vi "Tourner_Gyros.vi"(8 "Right":dbl, 9 "Left":dbl, 11 "Angle Voulu":dbl) -> (2 "Angle Reel":dbl)   [LabVIEW 2015]
uses:
  <vilib>/Rock Robotics/WPI/Utilities/WPI_GetSetVariantRefNum.vi
  <vilib>/Rock Robotics/Network Tables/NT Write Number.vi
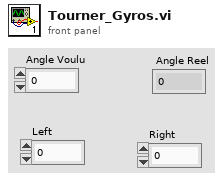
[diagram p1: front panel]
types:
  T1 = typedef "WPI_GyroDevRef.ctl" = cluster{"DevStatus":errorcluster, "Analog Channel":T2, "Offset":dbl, "Gain (VoltsPerDegree/Second)":dbl, "Gyro Type":enum16{"Analog", "XRS450"}, "Handle":i32, "SPI Bus":T3, "Device Found":bool, "Sample Rate":dbl, "Calibrate On Open":bool}
  T2 = typedef "FPGA_AIChannel.ctl" = enum8{"AI 0", "AI 1", "AI 2", "AI 3", "AI MXP 0", "AI MXP 1", "AI MXP 2", "AI MXP 3", "Invalid"}
  T3 = typedef "spi_bus.ctl" = enum16{"SPI On-Board, CS0", "SPI On-Board, CS1", "SPI On-Board, CS2", "SPI On-Board, CS3", "SPI MXP", "Invalid"}
  T4 = typedef "WPI_RobotDriveDevRef.ctl" = cluster{"DevStatus":errorcluster, "Motors[]":T5[], "Square Inputs":bool, "Max Output":dbl}
  T5 = typedef "WPI_MotorControlDeviceRef.ctl" = cluster{"DeviceStatus":errorcluster, "Type":T6, "PWM":cluster{"PWM Channel":T7, "DeadBand":T8}, "CAN":cluster{"Device Number":u8, "Control Mode":T9, "Semaphore":T10, "Max Vout":dbl, "TalonSRX Control Mode":T11}, "Invert":bool}
  T6 = typedef "WPI_MotorControlType.ctl" = enum16{"PWM", "CAN", "CANTalonSRX"}
  T7 = typedef "FPGA_DIOPWMChannel.ctl" = enum8{"PWM 0", "PWM 1", "PWM 2", "PWM 3", "PWM 4", "PWM 5", "PWM 6", "PWM 7", "PWM 8", "PWM 9", "PWM MXP 0", "PWM MXP 1", "PWM MXP 2", "PWM MXP 3", "PWM MXP 4", "PWM MXP 5", "PWM MXP 6", "PWM MXP 7", "PWM MXP 8", "PWM MXP 9", "Invalid"}
  T8 = typedef "WPI_PWMDeadband.ctl" = cluster{"Name":string, "maxPositivePwm":i32, "minPositivePwm":i32, "centerPwm":i32, "maxNegativePwm":i32, "minNegativePwm":i32, "angularRange":u16}
  T9 = typedef "WPI_CANJaguar_ControlMode.ctl" = enum8{"Percent VBus", "Current", "Speed", "Position", "Voltage"}
  T10 = typedef "Semaphore RefNum" = refnum<k1>
  T11 = typedef "WPI_CANTalonSRX_APIControlMode.ctl" = enum8{"Percent VBus", "Speed", "Position", "Slave", "Unchanged / Invalid", "Voltage Compensation", "Current", "Motion Profile"}
  T12 = typedef "WPI_EncoderDevRef.ctl" = cluster{"DevStatus":errorcluster, "EncoderIndex":T13, "CounterIndex":T14, "DistancePerCount":dbl, "Decoding Type":T15}
  T13 = typedef "FPGA_EncoderIdx.ctl" = enum8{"Enc 0", "Enc 1", "Enc 2", "Enc 3", "Enc 4", "Enc 5", "Enc 6", "Enc 7", "Invalid"}
  T14 = typedef "FPGA_CounterCtrSystemIndex.ctl" = enum8{"Ctr 0", "Ctr 1", "Ctr 2", "Ctr 3", "Ctr 4", "Ctr 5", "Ctr 6", "Ctr 7", "Invalid"}
  T15 = typedef "WPI_EncoderType.ctl" = enum16{"1x", "2x", "4x"}
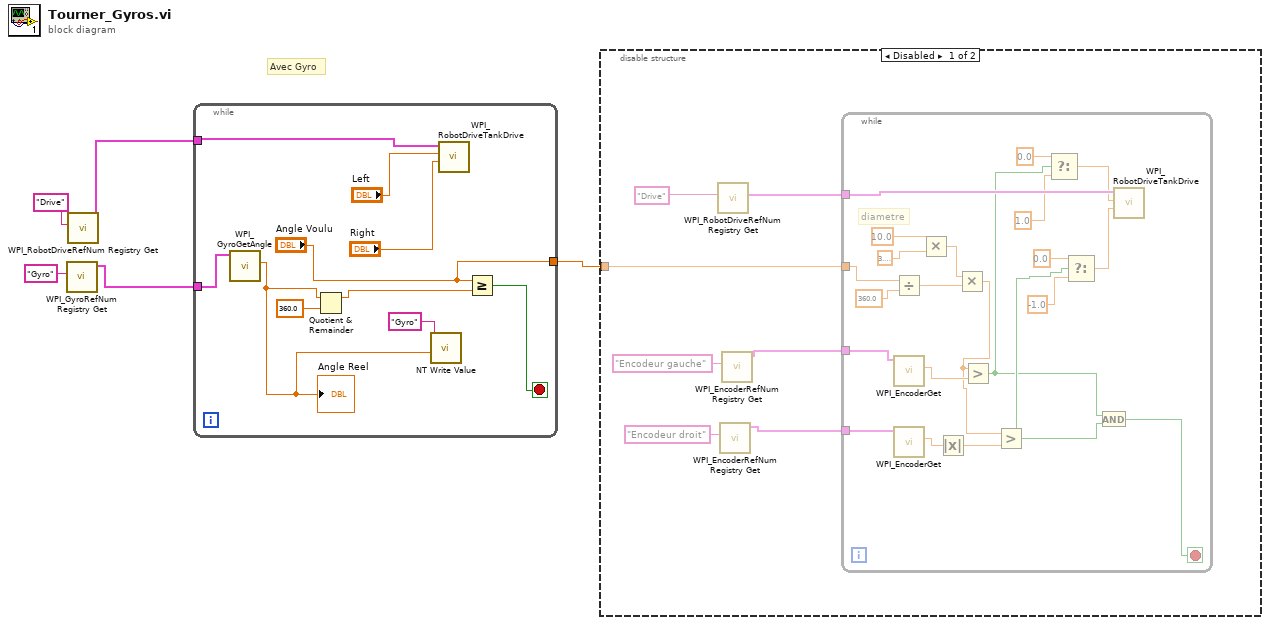
[diagram p0: block diagram]
diagram:
  # "Avec Gyro"
  n1 = call <vilib>:"WPI_GyroRefNum Registry Get.vi"("refnum name"="Gyro") -> ("GyroDevRef"=w3:T1)  [unwired: 9 in, 1 out]
  n2 = call <vilib>:"WPI_RobotDriveRefNum Registry Get.vi"("refnum name"="Drive") -> ("RobotDriveDevRef"=w4:T4)  [unwired: 9 in, 1 out]
  n3 = while {
    tunnel: w4 -> [w15]
    tunnel: w3 -> [w14]
    tunnel: ["Angle Voulu"] -> w1
    stop <- w13 stop-if-true
    n4 = call <vilib>:"WPI_GyroGetAngle.vi"("GyroDevRef"=w14) -> ("Angle"=w8:dbl)  [unwired: 6 in, 4 out]
    "Angle Reel" <- w8
    n5 = Quotient & Remainder(x=w8, y=360.0) -> (x-y*floor(x/y)=w11:dbl)  [unwired: 1 out]
    n6 = call-poly <vilib>:"NT Write Value.vi"("Numeric"=w8, "Name"="Gyro") -> ()  [unwired: 9 in, 1 out]
    n7 = call <vilib>:"WPI_RobotDriveTankDrive.vi"("Right axis value"="Right", "Left axis value"="Left", "RobotDriveDevRef"=w15) -> ()  [unwired: 6 in, 3 out]
    n8 = Greater Or Equal?(x="Angle Voulu", y=w11) -> (x >= y?=w13:bool)
  }
  n9 = disable-structure shown="Disabled" {
    disable-tunnel: w1 -> [w16 _]
    frame Disabled {
      n10 = call <vilib>:"WPI_RobotDriveRefNum Registry Get.vi"("refnum name"="Drive") -> ("RobotDriveDevRef"=w21:T4)  [unwired: 9 in, 1 out]
      n11 = call <vilib>:"WPI_EncoderRefNum Registry Get.vi"("refnum name"="Encodeur droit") -> ("EncoderDevRef"=w20:T12)  [unwired: 9 in, 1 out]
      n12 = call <vilib>:"WPI_EncoderRefNum Registry Get.vi"("refnum name"="Encodeur gauche") -> ("EncoderDevRef"=w19:T12)  [unwired: 9 in, 1 out]
      n13 = while {
        tunnel: w21 -> [w44]
        tunnel: w20 -> [w43]
        tunnel: w19 -> [w42]
        tunnel: w16 -> [w41]
        stop <- w31 stop-if-true
        # "diametre"
        n14 = Divide(x=w41, y=360.0) -> (x/y=w39:dbl)
        n15 = call <vilib>:"WPI_EncoderGet.vi"("EncoderDevRef"=w42) -> ("Distance"=w35:dbl)  [unwired: 5 in, 5 out]
        n16 = call <vilib>:"WPI_EncoderGet.vi"("EncoderDevRef"=w43) -> ("Distance"=w33:dbl)  [unwired: 5 in, 5 out]
        n17 = Multiply(x=10.0, y=3.141592653589793) -> (x*y=w37:dbl)
        n18 = Absolute Value(x=w33) -> (abs(x)=w32:dbl)
        n19 = Multiply(x=w37, y=w39) -> (x*y=w34:dbl)
        n20 = Greater?(x=w34, y=w35) -> (0:w24:bool)
        n21 = Greater?(x=w34, y=w32) -> (0:w28:bool)
        n22 = Select(t=0.0, s=w24, f=1.0 ("Left axis value")) -> (s? t:f=w23:dbl)
        n23 = Select(t=0.0, s=w28, f=-1.0 ("Right axis value")) -> (s? t:f=w27:dbl)
        n24 = And(x=w24, y=w28) -> (x .and. y?=w31:bool)
        n25 = call <vilib>:"WPI_RobotDriveTankDrive.vi"("Right axis value"=w27, "Left axis value"=w23, "RobotDriveDevRef"=w44) -> ()  [unwired: 6 in, 3 out]
      }
    }
    frame Enabled {
    }
  }
